vi "Wait(sec) text out.vi"(1 "extra wait (sec)":i32 min=0) -> (0 "Command text":string[][](array[string]))   [LabVIEW 2021]
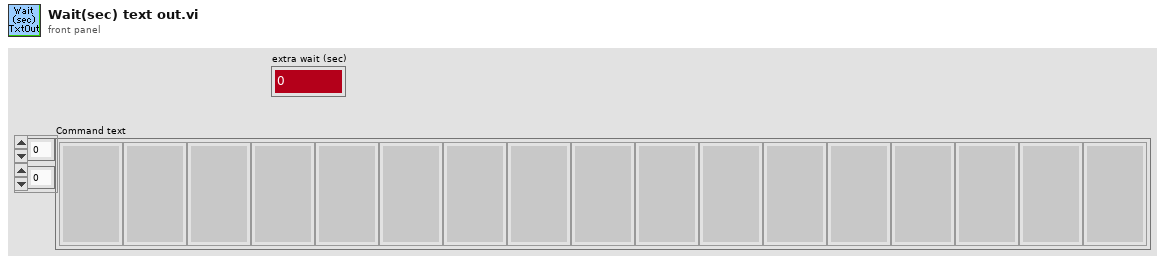
[diagram p1: front panel]
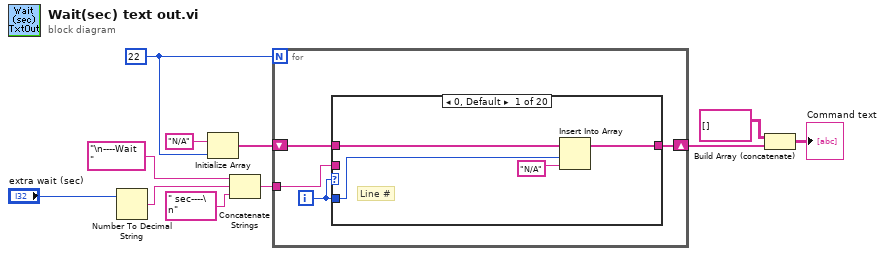
[diagram p0: block diagram]
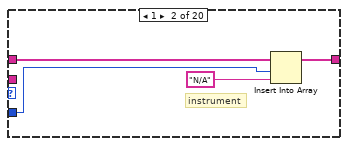
[diagram p2: hidden frame]
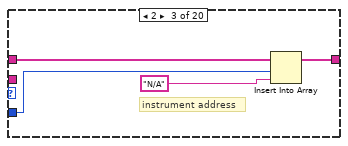
[diagram p3: hidden frame]
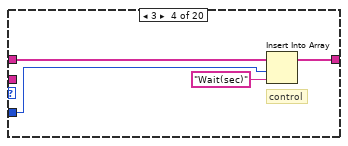
[diagram p4: hidden frame]
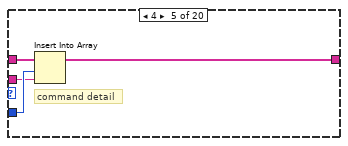
[diagram p5: hidden frame]
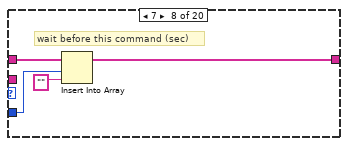
[diagram p8: hidden frame]
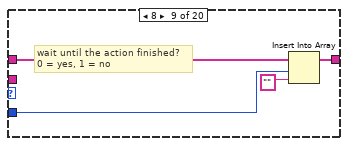
[diagram p9: hidden frame]
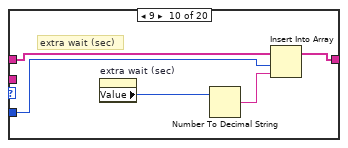
[diagram p10: hidden frame]
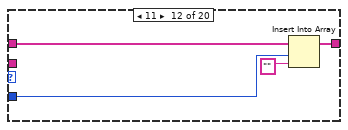
[diagram p12: hidden frame]
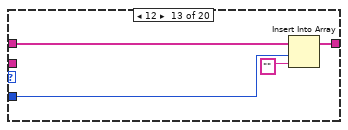
[diagram p13: hidden frame]
diagram:
  w9 = 22
  n1 = Number To Decimal String(number="extra wait (sec)") -> (decimal integer string=w2:string)  [unwired: 1 in]
  n2 = Initialize Array("N/A", w9) -> (w8:string[])
  n3 = Concatenate Strings("\n----Wait  " ("string"), w2, " sec----\n" ("string")) -> (w7:string)
  n4 = for {
    N: w9 -> [_]
    shift-right: [w12] -> w5
    shift-left: w8 -> [w14]
    tunnel: w7 -> [w13]
    i -> [w15]
    n5 = case shown="0, Default" w15 {
      tunnel: w15 -> [w18 w22 w26 w29 w34 _ _ w39 w43 w48 _ w53 w57 _ _ _ _ _ _ _]
      tunnel: w14 -> [w19 w21 w25 w30 w35 w36 w37 w41 w45 w50 w51 w54 w59 w60 w61 w62 w63 w64 w65 w66]
      tunnel: w13 -> [_ _ _ _ w33 _ _ _ _ _ _ _ _ _ _ _ _ _ _ _]
      tunnel: [w16 w20 w24 w28 w32 w36 w37 w40 w44 w49 w51 w55 w58 w60 w61 w62 w63 w64 w65 w66] -> w12
      frame 0, Default {
        # "Line #"
        n6 = Insert Into Array(array=w19, index=w18, new element="N/A") -> (w16:string[])
      }
      frame 1 {
        # "instrument"
        n7 = Insert Into Array(array=w21, index=w22, new element="N/A") -> (w20:string[])
      }
      frame 2 {
        # "instrument address"
        n8 = Insert Into Array(array=w25, index=w26, new element="N/A") -> (w24:string[])
      }
      frame 3 {
        # "control"
        n9 = Insert Into Array(array=w30, index=w29, new element="Wait(sec)") -> (w28:string[])
      }
      frame 4 {
        # "command detail"
        n10 = Insert Into Array(array=w35, index=w34, new element=w33) -> (w32:string[])
      }
      frame 5 {
        # "in  case 1"
      }
      frame 6 {
        # "in case 2"
      }
      frame 7 {
        # "wait before this command (sec)"
        n11 = Insert Into Array(array=w41, index=w39, new element="" ("new element/subarray")) -> (w40:string[])
      }
      frame 8 {
        # "wait until the action finished?\n0 = yes, 1 = no"
        n12 = Insert Into Array(array=w45, index=w43, new element="" ("new element/subarray")) -> (w44:string[])
      }
      frame 9 {
        # "extra wait (sec)"
        n13 = property on="extra wait (sec)" class="DigNum (strict)"() -> ("Value"=w47:i32)  [unwired: 2 in, 2 out]
        n14 = Number To Decimal String(number=w47) -> (decimal integer string=w46:string)  [unwired: 1 in]
        n15 = Insert Into Array(array=w50, index=w48, new element=w46) -> (w49:string[])
      }
      frame 10 {
      }
      frame 11 {
        n16 = Insert Into Array(array=w54, index=w53, new element="" ("new element/subarray")) -> (w55:string[])
      }
      frame 12 {
        n17 = Insert Into Array(array=w59, index=w57, new element="" ("new element/subarray")) -> (w58:string[])
      }
      frame 13 {
      }
      frame 14 {
      }
      frame 15 {
      }
      frame 16 {
      }
      frame 17 {
      }
      frame 18 {
      }
      frame 19 {
      }
    }
  }
  n18 = Build Array (concatenate)(string[][] [], w5) -> (→"Command text":string[][])
